vi "test device name mismatch error.vi"(8 "error in (no error)":errorcluster, 11 "TestCase in":refnum<class "Common System Tests.lvclass">) -> (0 "error out":errorcluster, 3 "TestCase out":refnum<class "Common System Tests.lvclass">)   [LabVIEW 2020, in "Common System Tests.lvclass"]
uses:
  Common System Tests.lvclass
  <vilib>/addons/_JKI Toolkits/VI Tester/TestCase.llb/TestCase.lvclass
  C:/Program Files (x86)/National Instruments/LabVIEW 2020/vi.lib/addons/_JKI Toolkits/VI Tester/TestCase.llb/TestCase.lvclass
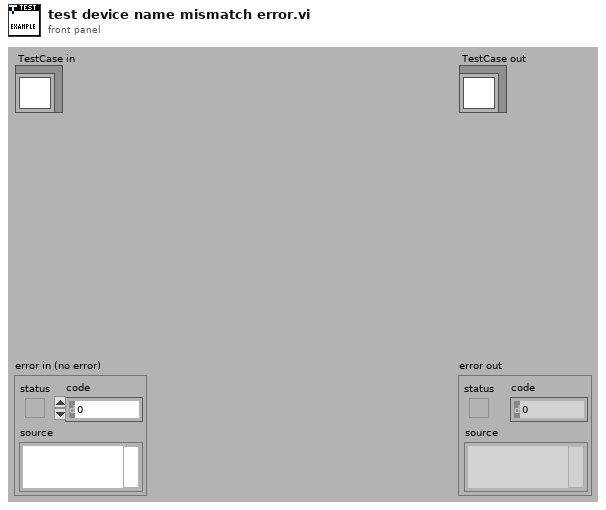
[diagram p1: front panel]
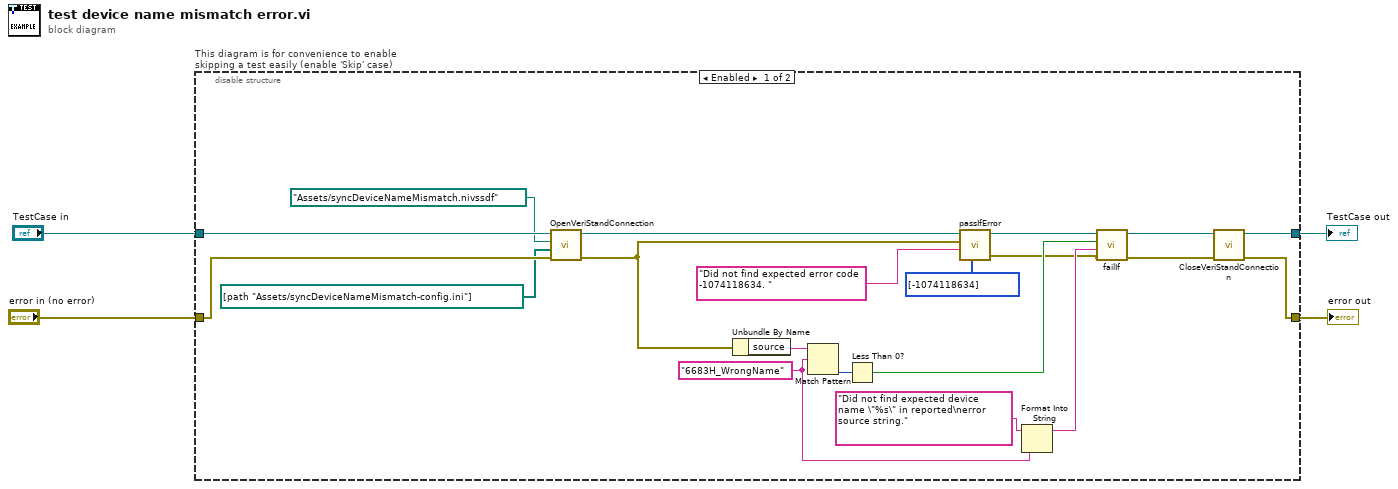
[diagram p0: block diagram]
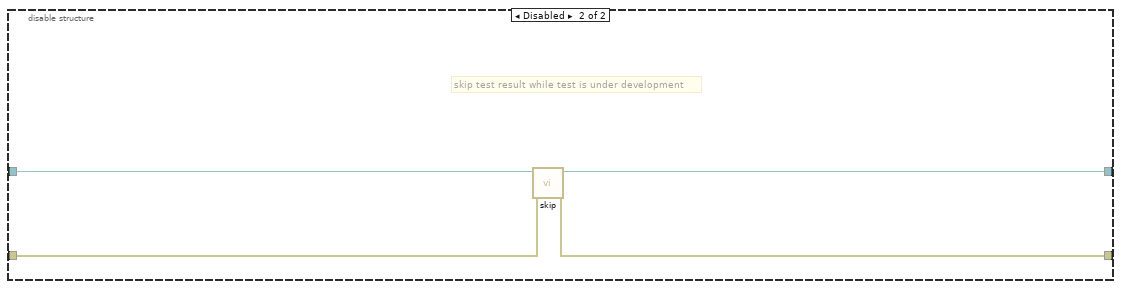
[diagram p2: hidden frame]
diagram:
  n1 = disable-structure "This diagram is for convenience to enable skipping a test easily (enable 'Skip' case)" shown="Enabled" {
    disable-tunnel: "TestCase in" -> [w24 w28]
    disable-tunnel: [w16 w26] -> w1
    disable-tunnel: [w15 w27] -> w3
    disable-tunnel: "error in (no error)" -> [w23 w25]
    frame Enabled {
      w18 = "6683H_WrongName" ("regular expression")
      n2 = call-dynamic "OpenVeriStandConnection.vi"("error in (no error)"=w23, "overrides files"=path[] [path "Assets/syncDeviceNameMismatch-config.ini"], "System Definition File"=path "Assets/syncDeviceNameMismatch.nivssdf", "VeriStand Test Case in"=w24) -> ("error out"=w6:errorcluster, "VeriStand Test Case out"=w21:refnum<class "Common System Tests.lvclass">)  [unwired: 5 in, 1 out]
      n3 = Unbundle By Name(w6) -> ("source"=w19:string)
      n4 = Match Pattern(string=w19, regular expression=w18) -> (offset past match=w10:i32)  [unwired: 1 in, 3 out]
      n5 = Less Than 0?(x=w10) -> (x < 0?=w9:bool)
      n6 = call-dynamic "passIfError.vi"("passing error codes (default = any error code)"=i32[] [-1074118634], "task (\"\")"="Did not find expected error code -1074118634. ", "error"=w6, "TestCase in"=w21) -> ("error out"=w7:errorcluster, "TestCase out"=w13:refnum<class "Common System Tests.lvclass">)  [unwired: 6 in]
      n7 = Format Into String(format string="Did not find expected device name \"%s\" in reported\nerror source string.", w18) -> (resulting string=w11:string)  [unwired: 2 in, 1 out]
      n8 = call-dynamic "failIf.vi"("error in (no error)"=w7, "message (\"\")"=w11, "fail"=w9, "TestCase in"=w13) -> ("error out"=w8:errorcluster, "TestCase out"=w12:refnum<class "Common System Tests.lvclass">)  [unwired: 6 in]
      n9 = call-dynamic "CloseVeriStandConnection.vi"("error in (no error)"=w8, "VeriStand Test Case in"=w12) -> ("error out"=w15:errorcluster, "VeriStand Test Case out"=w16:refnum<class "Common System Tests.lvclass">)  [unwired: 8 in]
    }
    frame Disabled {
      # "skip test result while test is under development"
      n10 = call <vilib>:"skip.vi"("error in (no error)"=w25, "TestCase in"=w28) -> ("error out"=w27:errorcluster, "TestCase out"=w26:refnum<class "Common System Tests.lvclass">)  [unwired: 8 in]
    }
  }
  "error out" <- w3
  "TestCase out" <- w1
